vi "solar_voy_def Find Packet (ID).vi"(6 "CMD":enum8{"CMD", "TLM"}(ring), 9 "ID":u16, 10 "PACKETS":T1[](array[typedef]) {"last_time" format="%<%H:%M:%S%3u %m/%d/%y>T"}) -> (2 "Index":i32)   [LabVIEW 2018]
doc: "This searches for a packet by ID."
uses:
  solar_voy_def_ctl ITEM TYPE.ctl
  type/solar_type Item Type.ctl
  solar_voy_def_ctl ITEM.ctl
  solar_voy_def_ctl PACKET_ID.ctl
  solar_voy_def_ctl PACKET.ctl
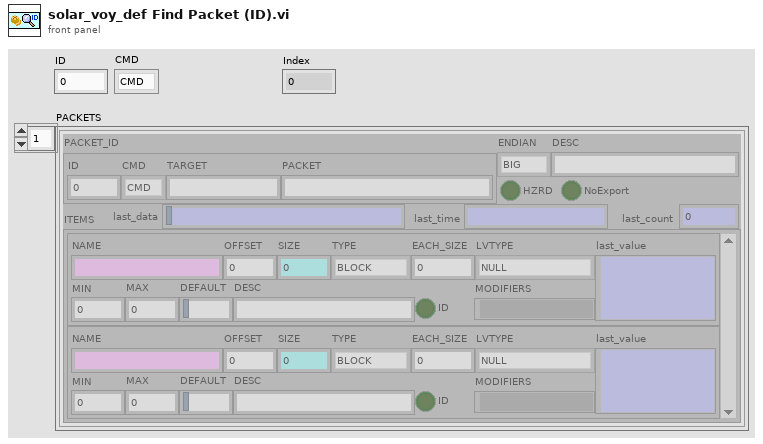
[diagram p1: front panel]
types:
  T1 = typedef "solar_voy_def_ctl PACKET.ctl" = cluster{"PACKET_ID":T2, "ENDIAN":enum8{"BIG", "LITTLE"}, "DESC":string, "HZRD":bool, "ITEMS":T3[], "NoExport":bool, "last_time":timestamp, "last_count":u32, "last_data":string}
  T2 = typedef "solar_voy_def_ctl PACKET_ID.ctl" = cluster{"ID":u16, "CMD":enum8{"CMD", "TLM"}, "TARGET":string, "PACKET":string}
  T3 = typedef "solar_voy_def_ctl ITEM.ctl" = cluster{"NAME":string, "OFFSET":i32, "SIZE":i32, "TYPE":T4, "EACH_SIZE":i32, "LVTYPE":T5, "MIN":dbl, "MAX":dbl, "DEFAULT":string, "DESC":string, "ID":bool, "MODIFIERS":variant, "last_value":variant}
  T4 = typedef "solar_voy_def_ctl ITEM TYPE.ctl" = enum8{"BLOCK", "INT", "UINT", "FLOAT", "STRING"}
  T5 = typedef "solar_type Item Type.ctl" = enum16{"NULL", "UNKNOWN", "CLUSTER", "I8", "I16", "I32", "I64", "U8", "U16", "U32", "U64", "U8_ENUM", "U16_ENUM", "U32_ENUM", "SGL", "DBL", "BOOLEAN", "STRING", "PATH", "VISA", "TAG", "TIME", "I8_1D", "I16_1D", "I32_1D", "I64_1D", "U8_1D", "U16_1D", "U32_1D", "U64_1D", "U8_ENUM_1D", "U16_ENUM_1D", "U32_ENUM_1D", "SGL_1D", "DBL_1D", "BOOLEAN_1D", "STRING_1D", "PATH_1D", "VISA_1D", "TAG_1D", "TIME_1D", "I8_2D", "I16_2D", "I32_2D", "I64_2D", "U8_2D", "U16_2D", "U32_2D", "U64_2D", "U8_ENUM_2D", "U16_ENUM_2D", "U32_ENUM_2D", "SGL_2D", "DBL_2D", "BOOLEAN_2D", "STRING_2D", "PATH_2D", "VISA_2D", "TAG_2D", "TIME_2D"}
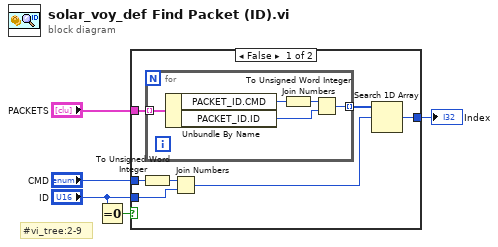
[diagram p0: block diagram]
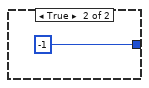
[diagram p2: hidden frame]
diagram:
  # "#vi_tree:2-9"
  n1 = Equal To 0?(x="ID") -> (x = 0?=w2:bool)
  n2 = case shown="False" w2 {
    tunnel: "PACKETS" -> [w12 _]
    tunnel: "ID" -> [w8 _]
    tunnel: [w11 -1 ("index of element")] -> w4
    tunnel: "CMD" -> [w9 _]
    frame False {
      n3 = To Unsigned Word Integer(number=w9) -> (unsigned 16bit integer=w7:u16)
      n4 = for {
        tunnel: w12 -> [w17] mode=indexing
        tunnel: [w13] -> w10 mode=indexing
        n5 = Unbundle By Name(w17) -> ("PACKET_ID.CMD"=w15:enum8{"CMD", "TLM"}, "PACKET_ID.ID"=w14:u16)
        n6 = To Unsigned Word Integer(number=w15) -> (unsigned 16bit integer=w16:u16)
        n7 = Join Numbers(hi=w16, lo=w14) -> ((hi.lo)=w13:u32)
      }
      n8 = Join Numbers(hi=w7, lo=w8) -> ((hi.lo)=w6:u32)
      n9 = Search 1D Array(1D array=w10, element=w6) -> (index of element=w11:i32)  [unwired: 1 in]
    }
    frame True {
    }
  }
  "Index" <- w4
